vi "write_param - test.vi"() -> ()   [LabVIEW 2014]
uses:
  FT_HMI.llb/GLOBAL_PUMPS_PARAMS.vi
  FT_HMI.llb/GLOBAL_GEN.vi
  ADS.llb/Global DIOs.vi
panel:
  in  "ST3_ETANCHEITE.TEMPS DE MESURE [s]":sgl
  in  "ST3_ETANCHEITE.TEMPS STABILISATION [s]":sgl
  in  "ST3_ETANCHEITE.TEMPS MISE SOUS PRESSION [s]":sgl
  in  "ST2_ASPIRATION.TEMPS DE MESURE PERTE [s]":sgl
  in  "ST2_ASPIRATION.TEMPS DE MESURE ASP [s]":sgl
  in  "ST2_ASPIRATION.STATUS CONTRE-PRESSION":bool
  in  "ST2_ASPIRATION.TEMPS POMPAGE [s]":sgl
  in  "ST1_HT.NO PROGRAMME":i32
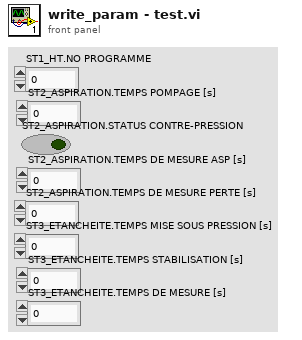
[diagram p1: front panel]
types:
  T1 = cluster{"GENERAL":cluster{"NO ARTICLE":string, "DESIGNATION":string, "TENSION [V]":sgl, "FREQUENCE [Hz]":sgl, "TYPE DEBIT":i8}, "ST1_HT":cluster{"STATUS HT":bool, "TENSION ISOLATION [V]":sgl, "COURANT ISOLATION [mA]":sgl, "TEMPS DE MESURE [s]":sgl, "NO PROGRAMME":i32}, "ST2_ASPIRATION":cluster{"STATUS H ASP":bool, "TEMPS POMPAGE [s]":sgl, "STATUS CONTRE-PRESSION":bool, "HAUTEUR ASPIRATION [m]":sgl, "TEMPS DE MESURE ASP [s]":sgl, "STATUS PERTE ASP":bool, "PERTE ASPIRATION [mbar]":sgl, "TEMPS DE MESURE PERTE [s] ":sgl}, "ST3_ETANCHEITE":cluster{"STATUS":bool, "ETANCHEITE [mbar]":sgl, "TEMPS MISE SOUS PRESSION [s]":sgl, "TEMPS STABILISATION [s]":sgl, "TEMPS DE MESURE [s]":sgl}, "ST4-5_DEBIT":cluster{"STATUS QMAX":bool, "GRAND DEBIT":bool, "PUMPING_TIME  [ms]":sgl, "DEBIT MIN [l/h]":sgl, "DEBIT MAX  [l/h]":sgl, "TEMPS DE MESURE QMAX [s]":sgl, "STATUS QTRAVAIL 1":bool, "DEBIT TRAVAIL 1 MIN [l/h]":sgl, "DEBIT TRAVAIL 1 MAX [l/h]":sgl, "PRESSION DE CONSIGNE 1 [bar]":sgl, "TEMPS DE REGLAGE PRESSION [s]":sgl, "TEMPS DE MESURE QTRAVAIL 1 [s]":sgl, "STATUS QTRAVAIL 2":bool, "DEBIT TRAVAIL 2 MIN [l/h]":sgl, "DEBIT TRAVAIL 2 MAX [l/h]":sgl, "PRESSION DE CONSIGNE 2 [bar]":sgl, "TEMPS DE MESURE QTRAVAIL 2 [s]":sgl, "STATUS CONSO":bool, "CONSOMMATION [A]":sgl, "TEMPS DE MESURE COURANT [s]":sgl}, "ST6_PRESSION":cluster{"STATUS PMAX":bool, "PUMPING TIME [s]":sgl, "PRESSION MIN [bar]":sgl, "TEMPS DE MESURE PMAX [s]":sgl, "STATUS PERTE PRESSION":bool, "PERTE PRESSION [mbar]":sgl, "TEMPS DE MESURE PERTE [s]":sgl}, "ST7_VIDANGE":cluster{"STATUS VIDANGE":bool, "TEMPS DE VIDANGE [S] ":sgl}, "ST8_IMPRESSION":cluster{"STATUS":bool, "ETIQUETTE":string}, "ST9_DECHARGEMENT":cluster{"STATUS":bool, "BOBINE A FIL":bool}, "DIVERS":cluster{"INDICE MODIF":string, "DATE MODIF":timestamp, "HISTORIQUE MODIF":string, "EMBOUT PRESSION":string, "EMBOUT ASPIRATION":string}}
  T2 = cluster{"ADS_GEN_GRAND_DEBIT_Header":i32, "ADS_ST1_HT_NO_PROG_Header":i32, "ADS_ST2_TEMPS_POMPAGE_Header":i32, "ADS_ST2_CONTRE_PRESSION_Header":i32, "ADS_ST2_TEMPS_MESURE_Header":i32, "ADS_ST2_TEMPS_MESURE_PERTE_PRESSION_Header":i32, "ADS_ST3_TEMPS_MISE_SOUS_PRESSION_Header":i32, "ADS_ST3_TEMPS_STABILISATION_Header":i32, "ADS_ST3_TEMPS_MESURE_Header":i32, "ADS_ST45_TEMPS_POMPAGE_Header":i32, "ADS_ST45_TEMPS_MESURE_DEBIT_MAX_Header":i32, "ADS_ST45_PRESSION_CONSIGNE_Header":i32, "ADS_ST45_TEMPS_REGLAGE_PRESSION_Header":i32, "ADS_ST45_TEMPS_MESURE_DEBIT_Header":i32, "ADS_ST6_TEMPS_POMPAGE_Header":i32, "ADS_ST6_TEMPS_MESURE_Header":i32, "ADS_ST6_TEMPS_MESURE_PERTE_PRESSION_Header":i32, "ADS_SAFETY_EM_State_Header":i32, "ADS_FLAGS_INIT_Header":i32, "ADS_FLAGS_AUTO_Header":i32, "ADS_FLAGS_SAFETY_Header":i32, "ADS_RESET_EMERGENCY_Header":i32, "ADS_PROG_STEPS_Header":i32, "ADS_ST1_HT_OK_Header":i32, "ADS_ST8_PRET_A_IMPRIMER_Header":i32, "ADS_ST8_IMPRESSION_OK_Header":i32, "ADS_ST2_VACUUM_Header":i32, "ADS_ST3_DELTA_P_Header":i32, "ADS_ST45_QMAX_Header":i32, "ADS_ST45_Q_Header":i32, "ADS_ST45_PRESSURE_Header":i32, "ADS_ST45_COURANT_Header":i32, "ADS_ST45_VACUUM_Header":i32, "ADS_ST5_MODE_VIDANGE_Header":i16, "ADS_ST45_POIDS_Header":i32, "ADS_GEMMA_Header":i32, "ADS_ST7_TEMPS_SECHAGE_Header":i32, "ADS_ST9_BOBINE_A_FIL_Header":i32}
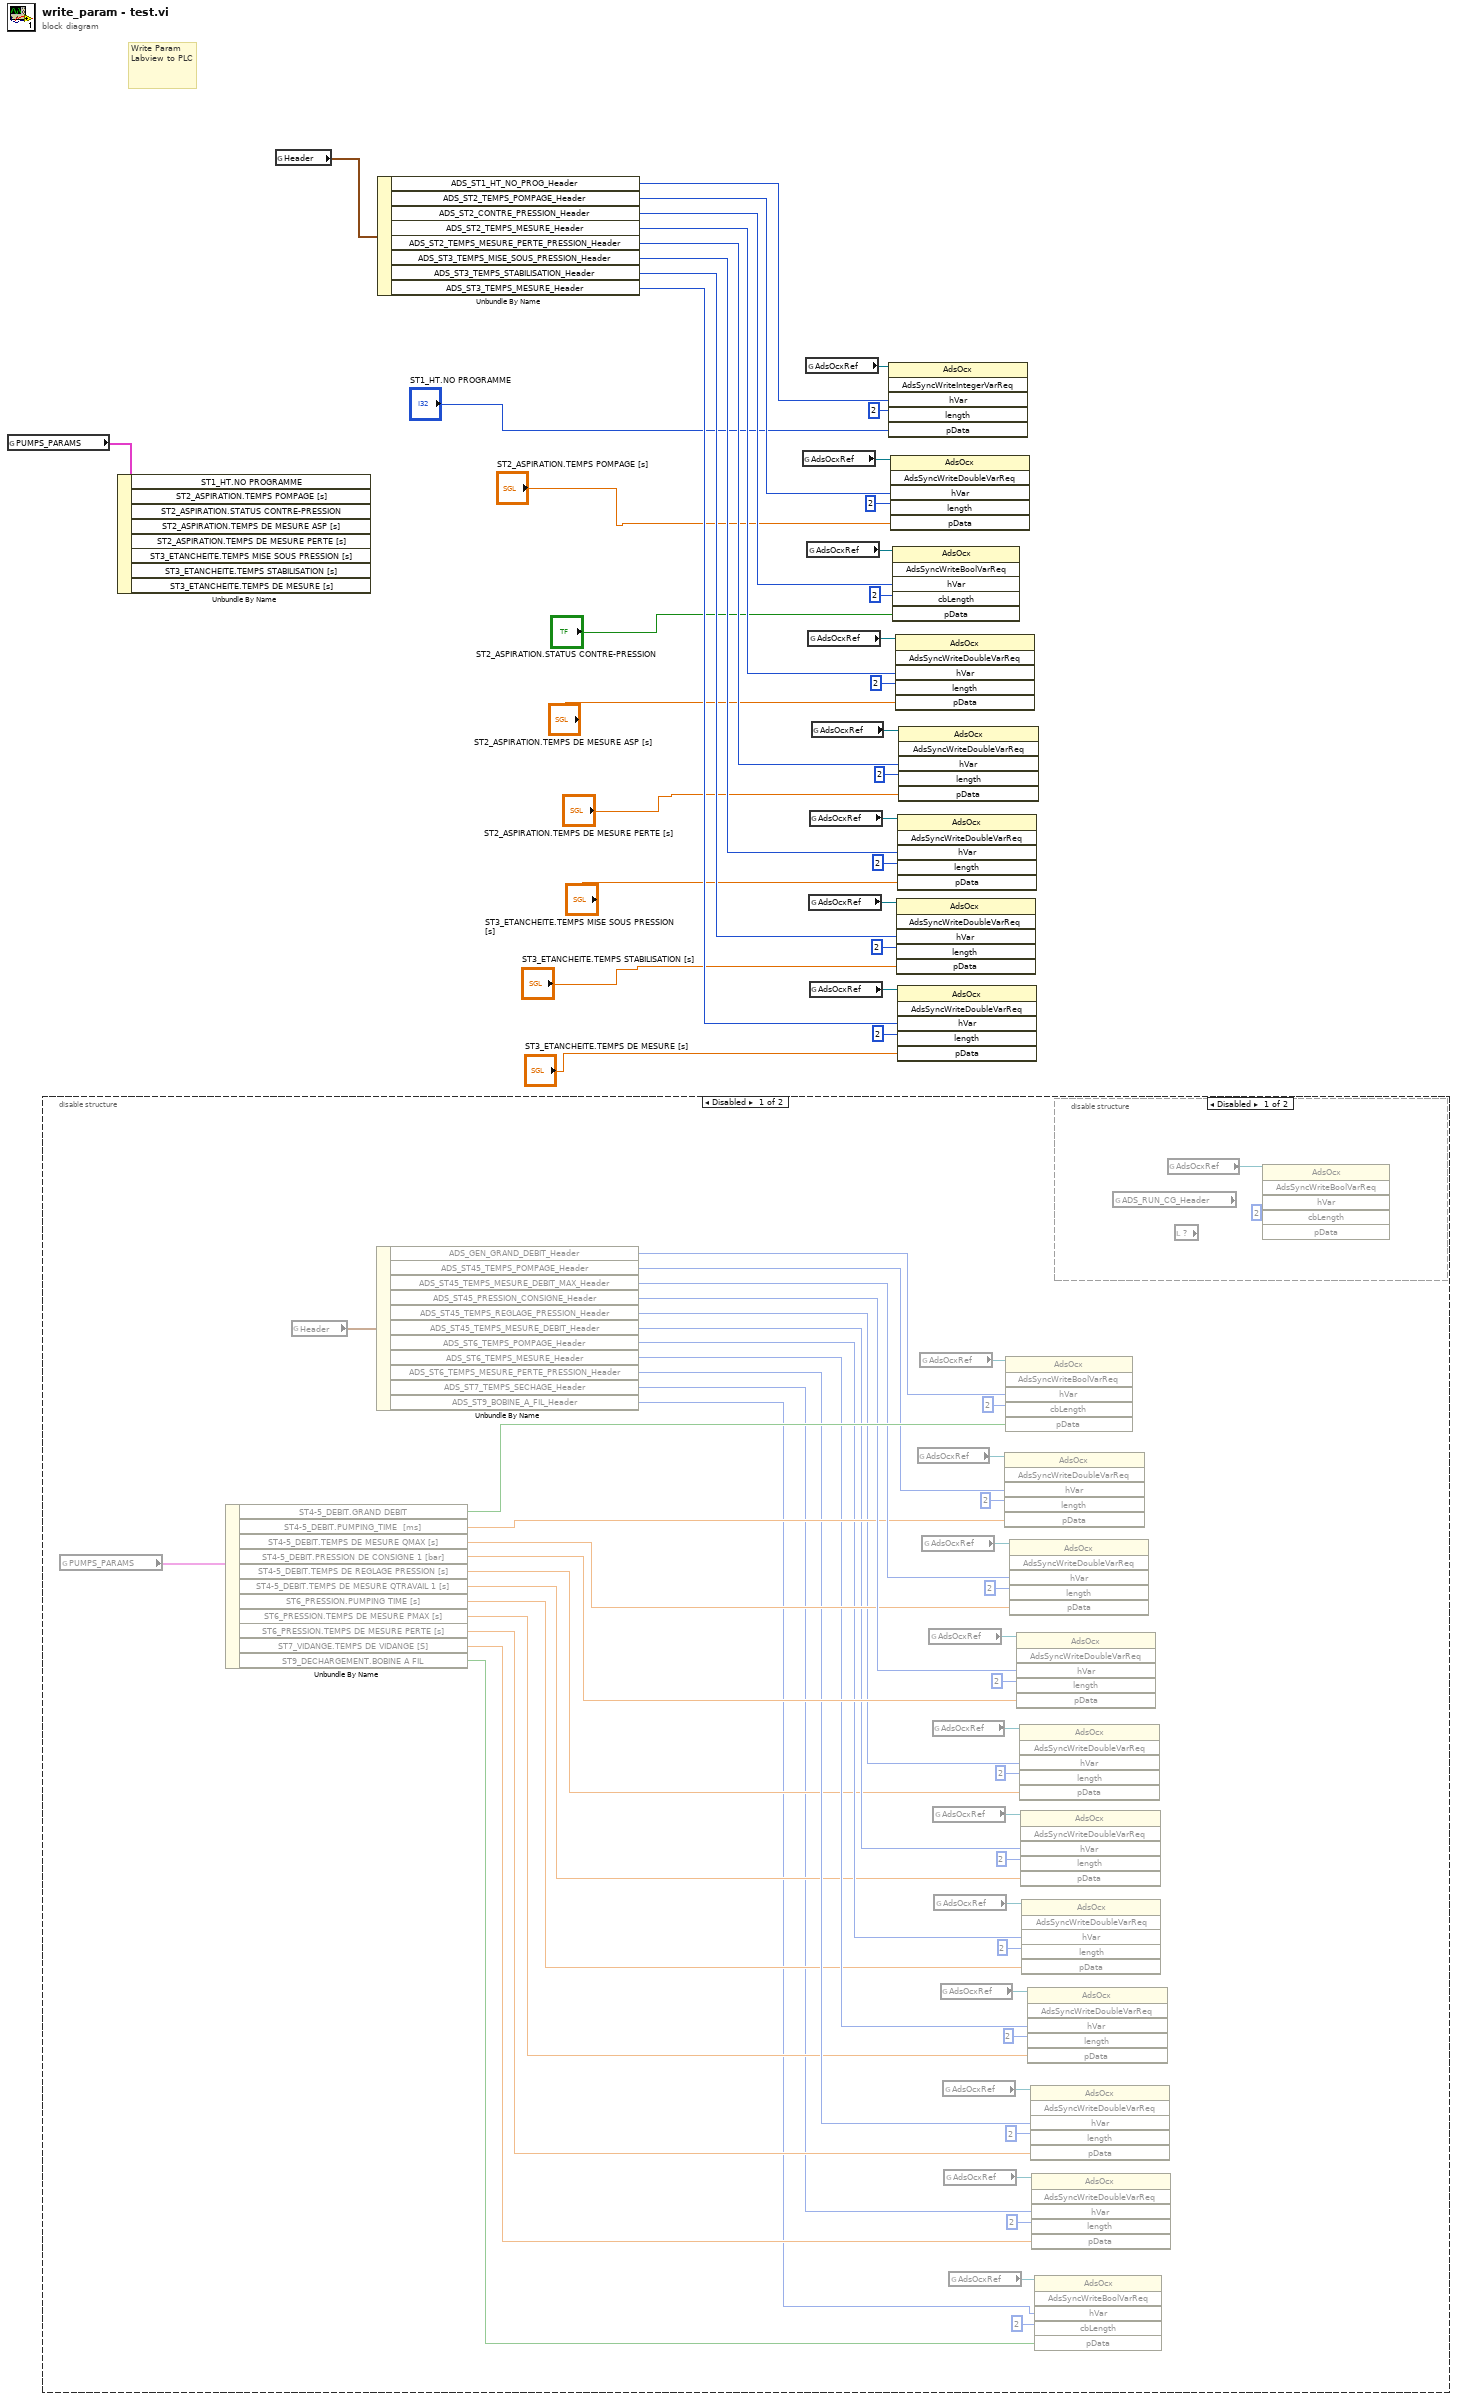
[diagram p0: block diagram]
diagram:
  # "Write Param Labview to PLC"
  n1 = global read "GLOBAL_PUMPS_PARAMS.vi" "PUMPS_PARAMS"() -> (w34:T1)
  n2 = disable-structure shown="Disabled" {
    frame Disabled {
      n3 = global read "GLOBAL_PUMPS_PARAMS.vi" "PUMPS_PARAMS"() -> (w80:T1)
      n4 = Unbundle By Name(w80) -> ("ST4-5_DEBIT.GRAND DEBIT"=w73:bool, "ST4-5_DEBIT.PUMPING_TIME  [ms]"=w58:sgl, "ST4-5_DEBIT.TEMPS DE MESURE QMAX [s]"=w57:sgl, "ST4-5_DEBIT.PRESSION DE CONSIGNE 1 [bar]"=w56:sgl, "ST4-5_DEBIT.TEMPS DE REGLAGE PRESSION [s]"=w47:sgl, "ST4-5_DEBIT.TEMPS DE MESURE QTRAVAIL 1 [s]"=w46:sgl, "ST6_PRESSION.PUMPING TIME [s]"=w45:sgl, "ST6_PRESSION.TEMPS DE MESURE PMAX [s]"=w44:sgl, "ST6_PRESSION.TEMPS DE MESURE PERTE [s]"=w42:sgl, "ST7_VIDANGE.TEMPS DE VIDANGE [S]"=w43:sgl, "ST9_DECHARGEMENT.BOBINE A FIL"=w41:bool)
      n5 = global read "Global DIOs.vi" "Header"() -> (w79:T2)
      n6 = Unbundle By Name(w79) -> ("ADS_GEN_GRAND_DEBIT_Header"=w74:i32, "ADS_ST45_TEMPS_POMPAGE_Header"=w72:i32, "ADS_ST45_TEMPS_MESURE_DEBIT_MAX_Header"=w60:i32, "ADS_ST45_PRESSION_CONSIGNE_Header"=w59:i32, "ADS_ST45_TEMPS_REGLAGE_PRESSION_Header"=w55:i32, "ADS_ST45_TEMPS_MESURE_DEBIT_Header"=w54:i32, "ADS_ST6_TEMPS_POMPAGE_Header"=w53:i32, "ADS_ST6_TEMPS_MESURE_Header"=w52:i32, "ADS_ST6_TEMPS_MESURE_PERTE_PRESSION_Header"=w48:i32, "ADS_ST7_TEMPS_SECHAGE_Header"=w39:i32, "ADS_ST9_BOBINE_A_FIL_Header"=w40:i32)
      n7 = global read "GLOBAL_GEN.vi" "AdsOcxRef"() -> (w77:refnum<k7>)
      n8 = global read "GLOBAL_GEN.vi" "AdsOcxRef"() -> (w75:refnum<k7>)
      n9 = global read "GLOBAL_GEN.vi" "AdsOcxRef"() -> (w70:refnum<k7>)
      n10 = global read "GLOBAL_GEN.vi" "AdsOcxRef"() -> (w68:refnum<k7>)
      n11 = global read "GLOBAL_GEN.vi" "AdsOcxRef"() -> (w66:refnum<k7>)
      n12 = global read "GLOBAL_GEN.vi" "AdsOcxRef"() -> (w64:refnum<k7>)
      n13 = global read "GLOBAL_GEN.vi" "AdsOcxRef"() -> (w63:refnum<k7>)
      n14 = global read "GLOBAL_GEN.vi" "AdsOcxRef"() -> (w61:refnum<k7>)
      n15 = global read "GLOBAL_GEN.vi" "AdsOcxRef"() -> (w49:refnum<k7>)
      n16 = global read "GLOBAL_GEN.vi" "AdsOcxRef"() -> (w38:refnum<k7>)
      n17 = global read "GLOBAL_GEN.vi" "AdsOcxRef"() -> (w35:refnum<k7>)
      n18 = invoke class="AdsOcx" method="AdsSyncWriteDoubleVarReq"(reference=w77, "hVar"=w72, "length"=2 ("phConnect"), "pData"=w58) -> ()  [unwired: 2 in, 6 out]
      n19 = invoke class="AdsOcx" method="AdsSyncWriteBoolVarReq"(reference=w75, "hVar"=w74, "cbLength"=2 ("phConnect"), "pData"=w73) -> ()  [unwired: 2 in, 6 out]
      n20 = invoke class="AdsOcx" method="AdsSyncWriteDoubleVarReq"(reference=w70, "hVar"=w60, "length"=2 ("phConnect"), "pData"=w57) -> ()  [unwired: 2 in, 6 out]
      n21 = invoke class="AdsOcx" method="AdsSyncWriteDoubleVarReq"(reference=w68, "hVar"=w59, "length"=2 ("phConnect"), "pData"=w56) -> ()  [unwired: 2 in, 6 out]
      n22 = invoke class="AdsOcx" method="AdsSyncWriteDoubleVarReq"(reference=w66, "hVar"=w55, "length"=2 ("phConnect"), "pData"=w47) -> ()  [unwired: 2 in, 6 out]
      n23 = invoke class="AdsOcx" method="AdsSyncWriteDoubleVarReq"(reference=w64, "hVar"=w54, "length"=2 ("phConnect"), "pData"=w46) -> ()  [unwired: 2 in, 6 out]
      n24 = invoke class="AdsOcx" method="AdsSyncWriteDoubleVarReq"(reference=w63, "hVar"=w53, "length"=2 ("phConnect"), "pData"=w45) -> ()  [unwired: 2 in, 6 out]
      n25 = invoke class="AdsOcx" method="AdsSyncWriteDoubleVarReq"(reference=w61, "hVar"=w52, "length"=2 ("phConnect"), "pData"=w44) -> ()  [unwired: 2 in, 6 out]
      n26 = invoke class="AdsOcx" method="AdsSyncWriteDoubleVarReq"(reference=w49, "hVar"=w48, "length"=2 ("phConnect"), "pData"=w42) -> ()  [unwired: 2 in, 6 out]
      n27 = invoke class="AdsOcx" method="AdsSyncWriteDoubleVarReq"(reference=w38, "hVar"=w39, "length"=2 ("phConnect"), "pData"=w43) -> ()  [unwired: 2 in, 6 out]
      n28 = invoke class="AdsOcx" method="AdsSyncWriteBoolVarReq"(reference=w35, "hVar"=w40, "cbLength"=2 ("phConnect"), "pData"=w41) -> ()  [unwired: 2 in, 6 out]
      n29 = disable-structure shown="Disabled" {
        frame Disabled {
          n30 = global read "Global DIOs.vi" "ADS_RUN_CG_Header"() -> ()  [unwired: 1 out]
          n31 = global read "GLOBAL_GEN.vi" "AdsOcxRef"() -> (w81:refnum<k7>)
          n32 = local read item#-1() -> ()  [unwired: 1 out]
          n33 = invoke class="AdsOcx" method="AdsSyncWriteBoolVarReq"(reference=w81, "cbLength"=2 ("phConnect")) -> ()  [unwired: 4 in, 6 out]
        }
        frame Enabled {
        }
      }
    }
    frame Enabled {
    }
  }
  n34 = Unbundle By Name(w34) -> ()  [unwired: 8 out]
  n35 = global read "Global DIOs.vi" "Header"() -> (w23:T2)
  n36 = Unbundle By Name(w23) -> ("ADS_ST1_HT_NO_PROG_Header"=w22:i32, "ADS_ST2_TEMPS_POMPAGE_Header"=w21:i32, "ADS_ST2_CONTRE_PRESSION_Header"=w20:i32, "ADS_ST2_TEMPS_MESURE_Header"=w19:i32, "ADS_ST2_TEMPS_MESURE_PERTE_PRESSION_Header"=w18:i32, "ADS_ST3_TEMPS_MISE_SOUS_PRESSION_Header"=w15:i32, "ADS_ST3_TEMPS_STABILISATION_Header"=w12:i32, "ADS_ST3_TEMPS_MESURE_Header"=w9:i32)
  n37 = global read "GLOBAL_GEN.vi" "AdsOcxRef"() -> (w30:refnum<k7>)
  n38 = global read "GLOBAL_GEN.vi" "AdsOcxRef"() -> (w32:refnum<k7>)
  n39 = global read "GLOBAL_GEN.vi" "AdsOcxRef"() -> (w28:refnum<k7>)
  n40 = global read "GLOBAL_GEN.vi" "AdsOcxRef"() -> (w26:refnum<k7>)
  n41 = global read "GLOBAL_GEN.vi" "AdsOcxRef"() -> (w13:refnum<k7>)
  n42 = global read "GLOBAL_GEN.vi" "AdsOcxRef"() -> (w16:refnum<k7>)
  n43 = global read "GLOBAL_GEN.vi" "AdsOcxRef"() -> (w10:refnum<k7>)
  n44 = global read "GLOBAL_GEN.vi" "AdsOcxRef"() -> (w24:refnum<k7>)
  n45 = invoke class="AdsOcx" method="AdsSyncWriteIntegerVarReq"(reference=w32, "hVar"=w22, "length"=2 ("phConnect"), "pData"="ST1_HT.NO PROGRAMME") -> ()  [unwired: 2 in, 6 out]
  n46 = invoke class="AdsOcx" method="AdsSyncWriteDoubleVarReq"(reference=w30, "hVar"=w21, "length"=2 ("phConnect"), "pData"="ST2_ASPIRATION.TEMPS POMPAGE [s]") -> ()  [unwired: 2 in, 6 out]
  n47 = invoke class="AdsOcx" method="AdsSyncWriteBoolVarReq"(reference=w28, "hVar"=w20, "cbLength"=2 ("phConnect"), "pData"="ST2_ASPIRATION.STATUS CONTRE-PRESSION") -> ()  [unwired: 2 in, 6 out]
  n48 = invoke class="AdsOcx" method="AdsSyncWriteDoubleVarReq"(reference=w26, "hVar"=w19, "length"=2 ("phConnect"), "pData"="ST2_ASPIRATION.TEMPS DE MESURE ASP [s]") -> ()  [unwired: 2 in, 6 out]
  n49 = invoke class="AdsOcx" method="AdsSyncWriteDoubleVarReq"(reference=w13, "hVar"=w12, "length"=2 ("phConnect"), "pData"="ST3_ETANCHEITE.TEMPS STABILISATION [s]") -> ()  [unwired: 2 in, 6 out]
  n50 = invoke class="AdsOcx" method="AdsSyncWriteDoubleVarReq"(reference=w16, "hVar"=w15, "length"=2 ("phConnect"), "pData"="ST3_ETANCHEITE.TEMPS MISE SOUS PRESSION [s]") -> ()  [unwired: 2 in, 6 out]
  n51 = invoke class="AdsOcx" method="AdsSyncWriteDoubleVarReq"(reference=w10, "hVar"=w9, "length"=2 ("phConnect"), "pData"="ST3_ETANCHEITE.TEMPS DE MESURE [s]") -> ()  [unwired: 2 in, 6 out]
  n52 = invoke class="AdsOcx" method="AdsSyncWriteDoubleVarReq"(reference=w24, "hVar"=w18, "length"=2 ("phConnect"), "pData"="ST2_ASPIRATION.TEMPS DE MESURE PERTE [s]") -> ()  [unwired: 2 in, 6 out]
